vi "Runner.vi"(8 "error in (no error)":errorcluster, 10 "Runnable":refnum<class "Runnable.lvclass">, 11 "Parallell Test Runner In":refnum<class "Parallel Test Runner.lvclass">) -> (0 "error out":errorcluster)   [LabVIEW 2020, in "Parallel Test Runner.lvclass"]
uses:
  Parallel Test Runner.lvclass
  Parallel Test Runner.lvclass/Parallel Test Runner.ctl
  LUnit Test Suite.lvclass
  Result Observer/Result Observer.lvclass
  Core/Result/Type.ctl
  Core/Result/Result.lvlib
  Core/Result/Status.ctl
  Core/Result/Result.ctl
  Execute Suite.vi
  Runnable.lvclass
  C:/git/astemes-lunit/source/LUnit Test Suite.lvclass
  C:/git/astemes-lunit/source/Runnable.lvclass
  C:/git/astemes-lunit/source/Framework/Parallel Test Runner/Parallel Test Runner.lvclass
  C:/git/astemes-lunit/source/Framework/Test Runner/Test Runner.lvclass
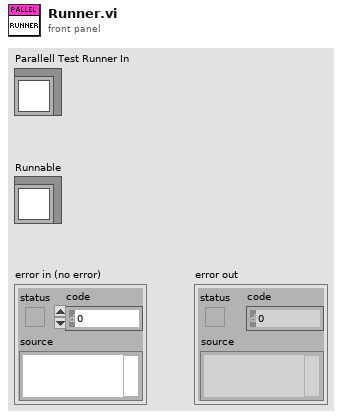
[diagram p1: front panel]
types:
  T1 = typedef "Result.lvlib/Result.ctl" = cluster{"Name":string, "Description":string, "Status":T2, "Result Type":T3, "Execution Time":dbl, "Data":cluster{"Expected":variant, "Actual":variant, "Delta":variant}}
  T2 = typedef "Result.lvlib/Status.ctl" = enum16{"", "Passed", "Failed", "Error", "Skipped", "Setup Error", "Broken", "Teardown Error"}
  T3 = typedef "Result.lvlib/Type.ctl" = enum16{"Test Case", "Test Suite", "Test Run", "Pass", "Fail", "Skip", "Pass if", "Fail if", "Pass if Error", "Fail if Error", "Pass if Equal", "Fail if Equal"}
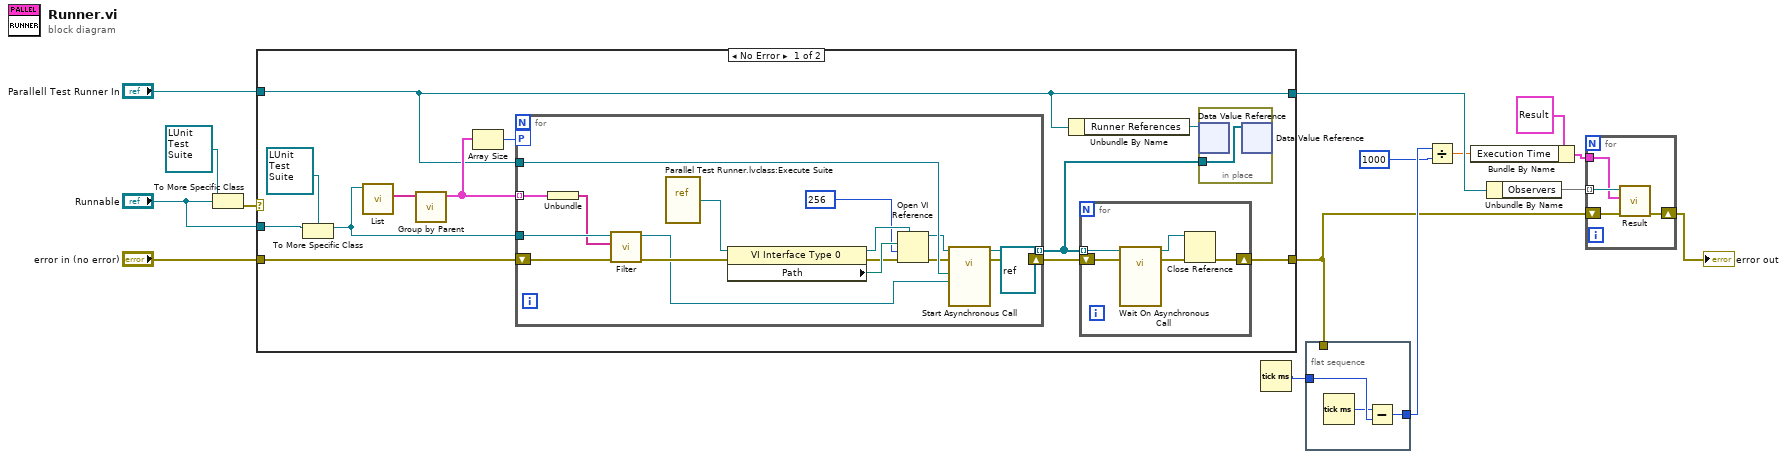
[diagram p0: block diagram]
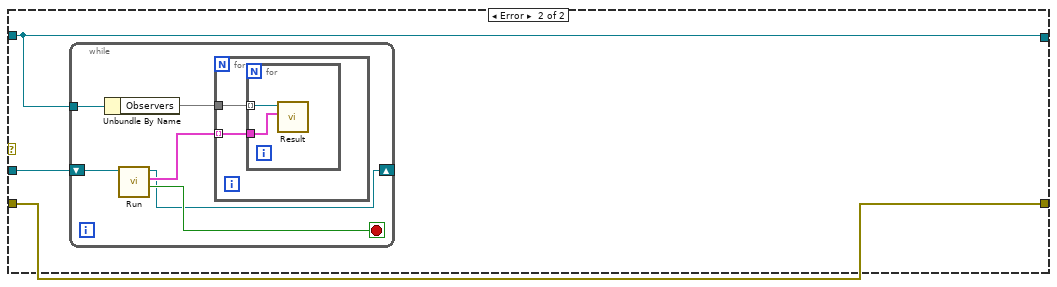
[diagram p2: hidden frame]
diagram:
  n1 = To More Specific Class(target class="Runnable", reference=refnum<class "LUnit Test Suite.lvclass"> refnum ("target class")) -> (error out=w9:errorcluster)  [unwired: 1 in, 1 out]
  n2 = case shown="No Error" w9 {
    tunnel: "Parallell Test Runner In" -> [w18 w52]
    tunnel: "error in (no error)" -> [w25 w50]
    tunnel: [w24 w50] -> w6
    tunnel: [w18 w52] -> w8
    tunnel: "Runnable" -> [w21 w51]
    frame No Error {
      n3 = To More Specific Class(target class=refnum<class "LUnit Test Suite.lvclass"> refnum, reference=w21) -> (specific class reference=w19:refnum<class "LUnit Test Suite.lvclass">)  [unwired: 1 in, 1 out]
      n4 = call "List.vi"("LUnit Test Suite In"=w19) -> ("List of Runnables"=w27:string[])  [unwired: 9 in, 1 out]
      n5 = call "Group by Parent.vi"("List of Runnables"=w27) -> ("Methods"=w23:cluster{"Methods":string[]}[])  [unwired: 10 in]
      n6 = Array Size(array=w23) -> (size(s)=w22:i32)
      n7 = for {
        tunnel: w19 -> [w44]
        shift-right: [w43] -> w26
        shift-left: w25 -> [w42]
        tunnel: w23 -> [w37] mode=indexing
        tunnel: [w39] -> w16 mode=indexing
        workers-P: w22 -> [_]
        tunnel: w18 -> [w38]
        (unwired) refnum<vi> refnum ("reference out")
        n8 = Unbundle(w37) -> ("Methods"=w36:string[])
        n9 = call "Filter.vi"("error in (no error)"=w42, "Selected Runnables"=w36, "LUnit Test Suite In"=w44) -> ("error out"=w41:errorcluster, "LUnit Test Suite Out"=w40:refnum<class "LUnit Test Suite.lvclass">)  [unwired: 7 in]
        n10 = vi-ref "Parallel Test Runner.lvclass:Execute Suite.vi"() -> (w35:refnum<vi>)
        n11 = property class="VI Interface Type 0"(reference=w35, error in=w41) -> (reference out=w33:refnum<vi>, error out=w32:errorcluster, "Path"=w34:path)
        n12 = Open VI Reference(type specifier VI Refnum (for type only)=w33, vi path=w34, options=256, error in (no error)=w32) -> (vi reference=w31:refnum<vi>, error out=w30:errorcluster)  [unwired: 2 in]
        n13 = call-by-ref "Start Asynchronous Call"(reference=w31, error in=w30, "Runnable"=w40, "Parallell Test Runner In"=w38) -> (reference out=w39:refnum<vi>, error out=w43:errorcluster)  [unwired: 10 in]
      }
      n14 = Unbundle By Name(w18) -> ("Runner References"=w17:refnum<data-value>)
      n15 = for {
        shift-right: [w48] -> w24
        shift-left: w26 -> [w49]
        tunnel: w16 -> [w47] mode=indexing
        n16 = call-by-ref "Wait On Asynchronous Call"(reference=w47, error in=w49) -> (reference out=w46:refnum<vi>, error out=w45:errorcluster)  [unwired: 12 in]
        n17 = Close Reference(reference=w46, error in (no error)=w45) -> (error out=w48:errorcluster)
      }
      n18 = in-place {
        in-place-border: w16 -> [w28]
        n19 = in-place-dvr #1(w17) -> ()  [unwired: 2 out]
        n20 = in-place-dvr #1(w28) -> ()  [unwired: 2 out]
      }
    }
    frame Error {
      n21 = while {
        shift-right: [w56] -> _
        shift-left: w51 -> [w55]
        tunnel: w52 -> [w54]
        stop <- w57 stop-if-true
        n22 = Unbundle By Name(w54) -> ("Observers"=w53:set{refnum<class "Result Observer.lvclass">})
        n23 = call-dynamic "Run.vi"("Runnable In"=w55) -> ("Done?"=w57:bool, "Results"=w58:T1[], "Runnable Out"=w56:refnum<class "Runnable.lvclass">)  [unwired: 7 in, 1 out]
        n24 = for {
          tunnel: w58 -> [w59] mode=indexing
          tunnel: w53 -> [w60]
          n25 = for {
            tunnel: w60 -> [w62] mode=indexing
            tunnel: w59 -> [w61]
            n26 = call-dynamic "Result.vi"("Result"=w61, "Result Observer In"=w62) -> ()  [unwired: 9 in, 1 out]
          }
        }
      }
    }
  }
  n27 = Tick Count (ms)() -> (millisecond timer value=w12:u32)
  n28 = flat-sequence {
    tunnel: w12 -> [w65]
    tunnel: [w64] -> w11
    tunnel: w6 -> [_]
    frame #0 {
      n29 = Tick Count (ms)() -> (millisecond timer value=w63:u32)
      n30 = Subtract(x=w63, y=w65) -> (x-y=w64:u32)
    }
  }
  n31 = Divide(x=w11, y=u32 1000) -> (x/y=w5:dbl)
  n32 = Bundle By Name(cluster=T1 {"Name"="", "Description"="", "Status"=enum."Passed", "Result Type"=enum."Test Run", "Execution Time"=0.0, "Data"={"Expected"=variant, "Actual"=variant, "Delta"=variant}} ("Result"), "Execution Time"=w5) -> (w2:T1)
  n33 = Unbundle By Name(w8) -> ("Observers"=w4:set{refnum<class "Result Observer.lvclass">})
  n34 = for {
    tunnel: w4 -> [w69] mode=indexing
    tunnel: w2 -> [w68]
    shift-right: [w66] -> w13
    shift-left: w6 -> [w67]
    n35 = call-dynamic "Result.vi"("error in (no error)"=w67, "Result"=w68, "Result Observer In"=w69) -> ("error out"=w66:errorcluster)  [unwired: 8 in]
  }
  "error out" <- w13
